vi "TDMS Write.vi"(7 "Channel Name":string, 8 "error in (no error)":errorcluster, 9 "Group Name":string, 10 "TDMS in":refnum<k34>, 11 "Variant in":refnum<class "Variant.lvclass">) -> (0 "error out":errorcluster, 2 "TDMS Out":refnum<k34>)   [LabVIEW 2020, in "Data.lvlib" / "Variant.lvclass"]
doc: "Write Generic Data to a TDMS file."
uses:
  Variant.lvclass
  Data.lvclass
  Generic Data.lvclass
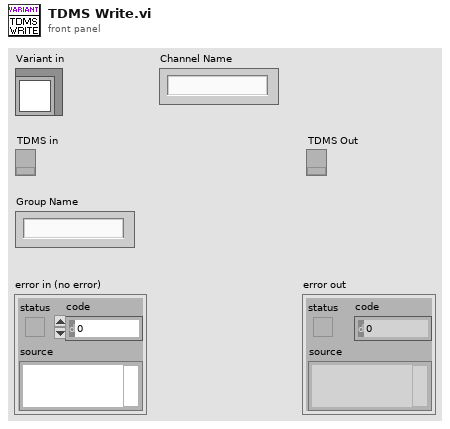
[diagram p1: front panel]
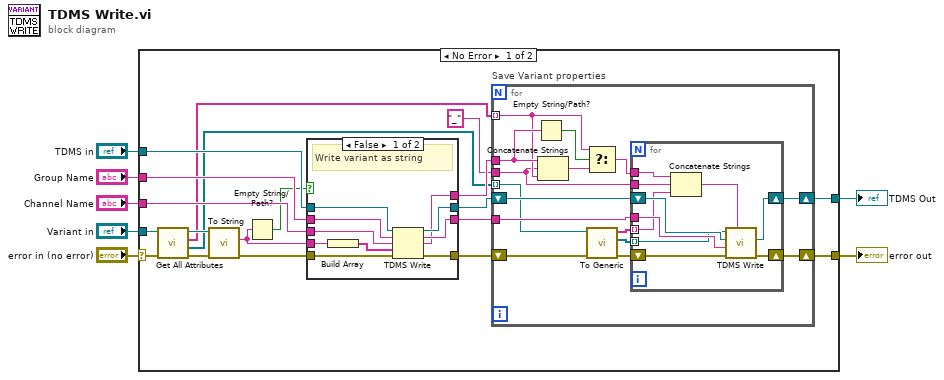
[diagram p0: block diagram]
diagram:
  n1 = case shown="No Error" "error in (no error)" {
    selector: "error in (no error)" -> [w17 w66]
    tunnel: [w11 w66] -> w1
    tunnel: "TDMS in" -> [w26 w67]
    tunnel: [w10 w67] -> w2
    tunnel: "Channel Name" -> [w25 _]
    tunnel: "Group Name" -> [w24 _]
    tunnel: "Variant in" -> [w18 _]
    frame No Error {
      n2 = call "Get All Attributes.vi"("error in (no error)"=w17, "Variant in"=w18) -> ("error out"=w19:errorcluster, "Data"=w9:refnum<class "Data.lvclass">[], "Names"=w16:string[], "Variant out"=w20:refnum<class "Variant.lvclass">)  [unwired: 6 in]
      n3 = call-dynamic "To String.vi"("error in (no error)"=w19, "Variant in"=w20) -> ("error out"=w23:errorcluster, "String"=w22:string)  [unwired: 8 in]
      n4 = Empty String/Path?(string/path=w22) -> (empty?=w21:bool)
      n5 = case shown="False" w21 {
        tunnel: [w61 w64] -> w12
        tunnel: w26 -> [w60 w65]
        tunnel: [w59 w65] -> w13
        tunnel: w25 -> [w58 w62]
        tunnel: w24 -> [w57 w63]
        tunnel: w23 -> [w55 w64]
        tunnel: w22 -> [w54 _]
        tunnel: [w53 w63] -> w15
        tunnel: [w52 w62] -> w14
        frame False {
          # "Write variant as string"
          n6 = Build Array(w54) -> (w56:string[])
          n7 = TDMS Write(0:w60, 5:w57, 7:w58, 9:w56, 11:w55) -> (4:w59:refnum<k34>, 6:w53:string, 8:w52:string, 15:w61:errorcluster)  [unwired: 1 in]
        }
        frame True {
          # "No Variant data"
        }
      }
      n8 = for "Save Variant properties" {
        tunnel: w16 -> [w38] mode=indexing
        tunnel: w15 -> [w41]
        tunnel: w14 -> [w39]
        shift-right: [w34] -> w10
        shift-left: w13 -> [w35]
        shift-right: [w33] -> w11
        shift-left: w12 -> [w31]
        tunnel: w9 -> [w32] mode=indexing
        tunnel: "_" ("string") -> [w29]
        n9 = Empty String/Path?(string/path=w39) -> (empty?=w40:bool)
        n10 = Concatenate Strings(w39, w29, w38) -> (w37:string)
        n11 = Select(t=w38, s=w40, f=w37) -> (s? t:f=w36:string)
        n12 = call-dynamic "To Generic.vi"("error in (no error)"=w31, "Data in"=w32) -> ("error out"=w30:errorcluster, "Generic Data"=w27:refnum<class "Generic Data.lvclass">[], "Data Name"=w28:string[])  [unwired: 7 in]
        n13 = for {
          tunnel: w41 -> [w51]
          tunnel: w36 -> [w50]
          tunnel: w29 -> [w45]
          shift-right: [w48] -> w34
          shift-left: w35 -> [w49]
          shift-right: [w47] -> w33
          shift-left: w30 -> [w44]
          tunnel: w28 -> [w43] mode=indexing
          tunnel: w27 -> [w42] mode=indexing
          n14 = Concatenate Strings(w50, w45, w43) -> (w46:string)
          n15 = call-dynamic "TDMS Write.vi"("Channel Name"=w46, "error in (no error)"=w44, "Group Name"=w51, "TDMS in"=w49, "Generic Data in"=w42) -> ("error out"=w47:errorcluster, "TDMS Out"=w48:refnum<k34>)  [unwired: 5 in]
        }
      }
    }
    frame Error {
    }
  }
  "error out" <- w1
  "TDMS Out" <- w2
